vi "Initialize Camera.vi"(8 "error in (no error)":errorcluster, 10 "handle index":u16, 11 "CCDCamera in":refnum<class "CCDCamera.lvclass">) -> (0 "error out":errorcluster, 3 "CCDCamera out":refnum<class "CCDCamera.lvclass">)   [LabVIEW 2018, in "CCDCamera.lvclass"]
uses:
  CCDCamera.lvclass
  C:/Users/observer/Desktop/SPARC4_ACS/SPARC4_ACS/Simulated_CCD_Camera/Simulated_CCD_Camera.lvclass
  Simulated_CCD_Camera/Simulated_CCD_Camera.lvclass
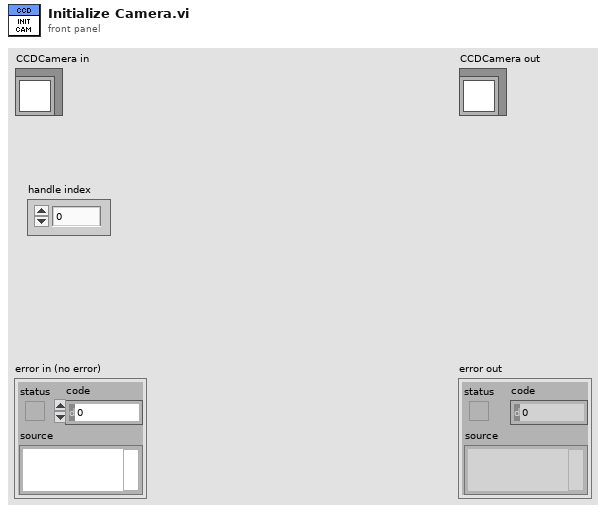
[diagram p1: front panel]
types:
  T1 = cluster{"CUBE_EXPOSURE_TIME":sgl, "CUBES_DONE":u16, "LAST_IMAGE_NAME":string, "DISK_SPACE":u16, "FRAMES_DONE":u16, "CCD_STATUS":string, "CURRENT_TEMPERATURE":i16, "TEMPERATURE_STATUS":string, "FRAME_EXPOSURE_TIME":u16, "CCD_ON_OFF":bool, "SERIAL_NUMBER":u16, "ACQUIRING":bool}
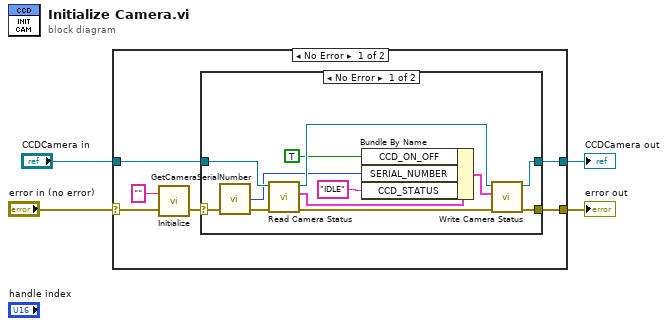
[diagram p0: block diagram]
diagram:
  n1 = case shown="No Error" "error in (no error)" {
    selector: "error in (no error)" -> [w9 w26]
    tunnel: [w7 w26] -> w1
    tunnel: [w8 w25] -> w2
    tunnel: "CCDCamera in" -> [w6 w25]
    frame No Error {
      n2 = call <userlib>:"Initialize.vi"("error in (no error)"=w9, "directory (\"\")"="" ("directory (\"\")")) -> ("error out"=w10:errorcluster)  [unwired: 1 out]
      n3 = case shown="No Error" w10 {
        selector: w10 -> [w21 w23]
        tunnel: w6 -> [w15 w24]
        tunnel: [w17 w24] -> w8
        tunnel: [w18 w23] -> w7
        frame No Error {
          n4 = call <userlib>:"GetCameraSerialNumber.vi"("error in (no error)"=w21) -> ("error out"=w20:errorcluster, "number"=w11:i32)  [unwired: 2 in, 1 out]
          n5 = call "Read Camera Status.vi"("error in (no error)"=w20, "CCDCamera in"=w15) -> ("error out"=w19:errorcluster, "Camera Status"=w14:T1, "CCDCamera out"=w16:refnum<class "CCDCamera.lvclass">)  [unwired: 7 in]
          n6 = Bundle By Name(cluster=w14, "CCD_ON_OFF"=TRUE ("Initialization"), "SERIAL_NUMBER"=w11, "CCD_STATUS"="IDLE" ("Camera Status.STATUS")) -> (w13:T1)
          n7 = call "Write Camera Status.vi"("error in (no error)"=w19, "Camera Status"=w13, "CCDCamera in"=w16) -> ("error out"=w18:errorcluster, "CCDCamera out"=w17:refnum<class "CCDCamera.lvclass">)  [unwired: 7 in]
        }
        frame Error {
        }
      }
    }
    frame Error {
    }
  }
  "error out" <- w1
  "CCDCamera out" <- w2
